vi "Get All Items.vi"(8 "error in (no error)":errorcluster, 11 "JSON Object in":refnum<class "JSON Object.lvclass">) -> (0 "error out":errorcluster, 1 "Values":refnum<class "JSON Value.lvclass">[](array[class]), 2 "Item Names":string[](array[string]), 3 "JSON Object out":refnum<class "JSON Object.lvclass">)   [LabVIEW 2011, in "JSON Object.lvclass"]
doc: "Returns the names of the Object's elements.\n\nCopyright 2012 James David Powell, Shaun Rumbell and Ton Plomp\nMore information on http://lavag.org/topic/16217-cr-json-labview"
uses:
  JSON Object.lvclass
  JSON Value/JSON Value.lvclass
  JSON Object.lvclass/JSON Object.ctl
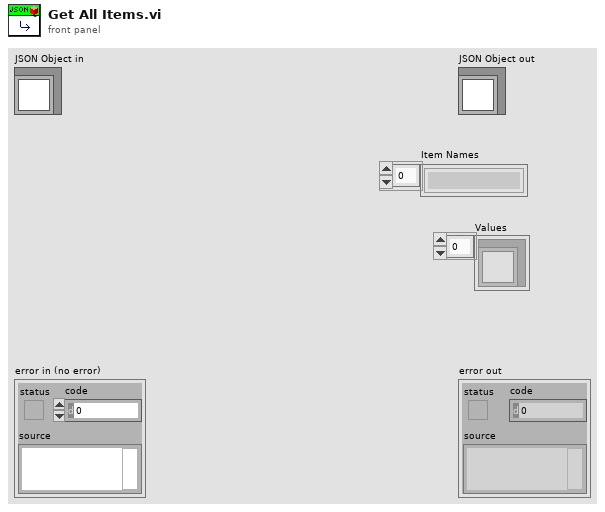
[diagram p1: front panel]
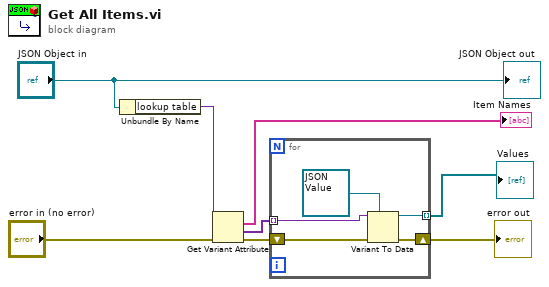
[diagram p0: block diagram]
diagram:
  n1 = Unbundle By Name("JSON Object in") -> ("lookup table"=w7:variant)
  n2 = Get Variant Attribute(Variant=w7, error in="error in (no error)") -> (names=→"Item Names":string[], values=w4:variant[], error out=w2:errorcluster)  [unwired: 2 in, 1 out]
  n3 = for {
    tunnel: w4 -> [w12] mode=indexing
    tunnel: [w11] -> w3 mode=indexing
    shift-right: [w9] -> w1
    shift-left: w2 -> [w10]
    n4 = Variant To Data(error in=w10, type=refnum<class "JSON Value.lvclass"> refnum ("JSON Value.lvclass"), Variant=w12) -> (data=w11:refnum<class "JSON Value.lvclass">, error out=w9:errorcluster)
  }
  "error out" <- w1
  "Values" <- w3
  "JSON Object out" <- "JSON Object in"
